vi "Multiline string updater.vi"(6 "Append to bottom":bool=TRUE, 9 "Lines to keep":u8, 10 "String to add":string, 11 "Multiline string in":string) -> (3 "Multiline string out":string)   [LabVIEW 2026, in "TALOS.lvlib" / "Father of all uServices.lvlib" / "Father of all uServices.lvclass"]
uses:
  Father of all uServices.lvclass
  <vilib>/AdvancedString/Delimited String to 1D String Array (string).vi
  <vilib>/AdvancedString/1D String Array to Delimited String (string).vi
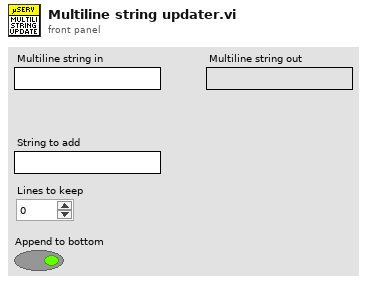
[diagram p1: front panel]
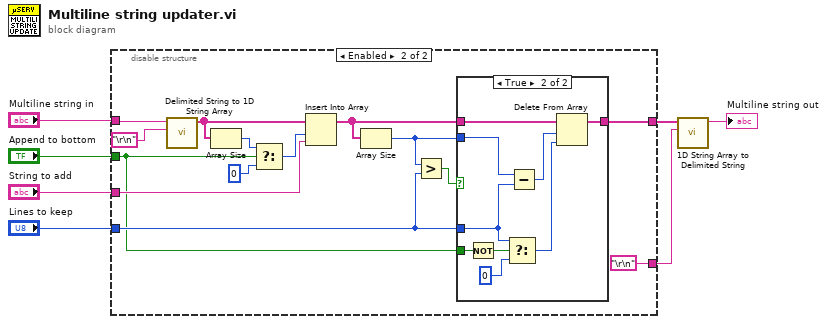
[diagram p0: block diagram]
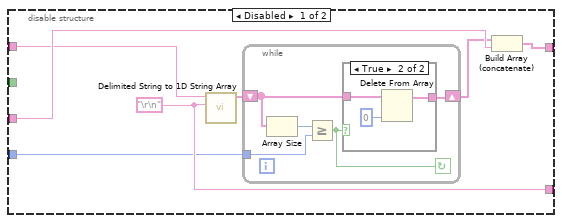
[diagram p2: hidden frame]
diagram:
  n1 = disable-structure shown="Enabled" {
    disable-tunnel: [w14 "\r\n"] -> w6
    disable-tunnel: [w13 w25] -> w5
    disable-tunnel: "String to add" -> [w12 w32]
    disable-tunnel: "Lines to keep" -> [w10 w28]
    disable-tunnel: "Multiline string in" -> [w8 w37]
    disable-tunnel: "Append to bottom" -> [_ w26]
    frame Disabled {
      w14 = "\r\n"
      n2 = call-poly <vilib>:"Delimited String to 1D String Array.vi"("delimiter"=w14, "delimited string"=w8) -> ("string array"=w9:string[])  [unwired: 9 in]
      n3 = while {
        tunnel: w10 -> [w18]
        shift-right: [w16] -> w11
        shift-left: w9 -> [w17]
        stop <- w15 continue-if-true
        n4 = Array Size(array=w17) -> (size(s)=w19:i32)
        n5 = Greater Or Equal?(x=w19, y=w18) -> (x >= y?=w15:bool)
        n6 = case shown="True" w15 {
          tunnel: w17 -> [w20 w23]
          tunnel: [w20 w21] -> w16
          frame False {
          }
          frame True {
            n7 = Delete From Array(array=w23, index=0) -> (array with subset deleted=w21:string[])  [unwired: 1 in, 1 out]
          }
        }
      }
      n8 = Build Array (concatenate)(w11, w12) -> (w13:string[])
    }
    frame Enabled {
      n9 = call-poly <vilib>:"Delimited String to 1D String Array.vi"("delimiter"="\r\n", "delimited string"=w37) -> ("string array"=w33:string[])  [unwired: 9 in]
      n10 = Array Size(array=w33) -> (size(s)=w35:i32)
      n11 = Select(t=w35, s=w26, f=0) -> (s? t:f=w27:i32)
      n12 = Insert Into Array(array=w33, index=w27, new element=w32) -> (w29:string[])
      n13 = Array Size(array=w29) -> (size(s)=w30:i32)
      n14 = Greater?(x=w30, y=w28) -> (0:w31:bool)
      n15 = case shown="True" w31 {
        tunnel: w30 -> [_ w46]
        tunnel: w29 -> [w38 w47]
        tunnel: w28 -> [_ w43]
        tunnel: w26 -> [_ w44]
        tunnel: [w38 w39] -> w25
        frame False {
        }
        frame True {
          n16 = Not(x=w44) -> (.not. x?=w40:bool)
          n17 = Select(t=w43, s=w40, f=u8 0) -> (s? t:f=w41:u8)
          n18 = Subtract(x=w46, y=w43) -> (x-y=w45:i32)
          n19 = Delete From Array(array=w47, length=w45, index=w41) -> (array with subset deleted=w39:string[])  [unwired: 1 out]
        }
      }
    }
  }
  n20 = call-poly <vilib>:"1D String Array to Delimited String.vi"("delimiter"=w6, "string array"=w5) -> ("delimited string"=→"Multiline string out":string)  [unwired: 9 in]
